vi "Main.vi"() -> ()   [LabVIEW 2019]
doc: "Main Program initialize config files, handles user inputs, image acquisition, object detection and image storing. User interface is handled in a state machine sending outputs."
uses:
  controls/State.ctl
  controls/Data.ctl
  <vilib>/userdefined/High Color/IMAQdx.ctl
  <vilib>/vision/Image Controls.llb/IMAQ Image.ctl
  b1a6e15a-21f6-4224-89c9-cebb1e441bce.vi
  4203ab90-da59-4329-829c-edbd02661f10.vi
  <extravilib>/ChannelInstances/Tag-bool/Read With Abort.vi
  <extravilib>/ChannelInstances/Tag-t'Data.ctl'/Read With Abort.vi
  <extravilib>/ChannelInstances/Tag-c(bool,bool)/Read With Abort.vi
  <extravilib>/ChannelInstances/Tag-c(bool,bool)/Write With Abort.vi
  <extravilib>/ChannelInstances/Tag-t'Data.ctl'/Write With Abort.vi
  <extravilib>/ChannelInstances/Tag-bool/Write With Abort.vi
  <extravilib>/ChannelInstances/Tag-c(bool,bool)/Instantiate.vi
  <extravilib>/ChannelInstances/Tag-t'Data.ctl'/Instantiate.vi
  <extravilib>/ChannelInstances/Tag-bool/Instantiate.vi
  <extravilib>/ChannelInstances/Tag-bool/EndpointRead.vi
  <extravilib>/ChannelInstances/Tag-t'Data.ctl'/EndpointRead.vi
  <extravilib>/ChannelInstances/Tag-c(bool,bool)/EndpointRead.vi
  <extravilib>/ChannelInstances/Tag-c(bool,bool)/Endpoint.vi
  <extravilib>/ChannelInstances/Tag-t'Data.ctl'/Endpoint.vi
  <extravilib>/ChannelInstances/Tag-bool/Endpoint.vi
  <extravilib>/ChannelInstances/Tag-bool.lvlib
  <extravilib>/ChannelInstances/Tag-t'Data.ctl'.lvlib
  <extravilib>/ChannelInstances/Tag-c(bool,bool).lvlib
panel:
  in  "Tab Control":T1(tab)
  in  "Exposure Time":dbl=1000.0
  in  "Exposure":enum32{"Item 0", "Item 1", "Item 2", "Item 3"}(radio)=enum."Item 3"
  in  "Aperture":enum32{"Item 0", "Item 1", "Item 2", "Item 3"}(radio)
  in  "Other notes":string caption="Sample Name"
  in  "Species Name":string="Test Sample" caption="Sample Name"
  in  "Station":string="Station" caption="Sample Name"
  in  "Collection date":string="24/06/2016" caption="Collection Date (DD/MM/YYYY)"
  out "Ready":bool
  in  "Operator":string="MRJ" caption="Sample Name"
  out "Active":bool
  in  "Start Image Capture":bool
  in  "Sample Name":string="#0000"
  in  "Stop Image Capture":bool
  in  "Calibration Pictures":bool
  out "Camera 2":bool
  out "Camear 1":bool
  out "Pump":bool
  out "Actuator":bool
  in  "Connect Systems":bool
  in  "Exit":bool
  in  "Empty and Refill":bool
  in  "Start System":bool
  in  "Empty System":bool
  out "Process queue":T2(graph)
  out "Image Saving":T2(graph)
  in  "Empty Cuvette":bool
  in  "Max large object threshold":i32=4 min=1
  in  "Change Crop":bool
  in  "DetectCrop":dbl=30.0 caption="Movement Detection size" format="%#_g %"
  in  "Sample size threshold":i32=500 min=1
  in  "New Sample timeout":i32=50 min=1
  out "Target framerate":i32=100
  in  "Light intensity":i32(slide)=100 min=1 max=100 scale=1.0..100.0 scale format="%.0f%"
  in  "Max Framerate":i32=100 min=1
  in  "Overload threshold":i32=50 min=1
  in  "Img Save Que Size":i32=100 caption="Image Save Queue Size" min=1
  in  "Img Proc Que Size":i32=200 caption="Image Processing Queue Size" min=1
  in  "Manual Close":bool
  in  "Manual Open":bool
  out "Current Position":string
  in  "Position":bool
  in  "Pump Cycle":bool
  in  "Pump Bottom":bool
  in  "Pump Top":bool
  in  "Pump Terminate":bool
  out "Framerate":i32 caption="Current Framerate"
  out "Camera 1":T3(plugin-control)
  out "Camera 2":T3(plugin-control)
  out "Camera 1 Detect":T3(plugin-control)
  out "Camera 2 Detect":T3(plugin-control)
  out "Camera 1 Binary":T3(plugin-control)
  out "Camera 2 Binary":T3(plugin-control)
  # "SRS Software - Version 1.2.0.1"
  # "Connections"
  # "Detection settings"
  # "Image capture settings"
  # "Buffer settings"
  # "Hatch control"
  # "Pump"
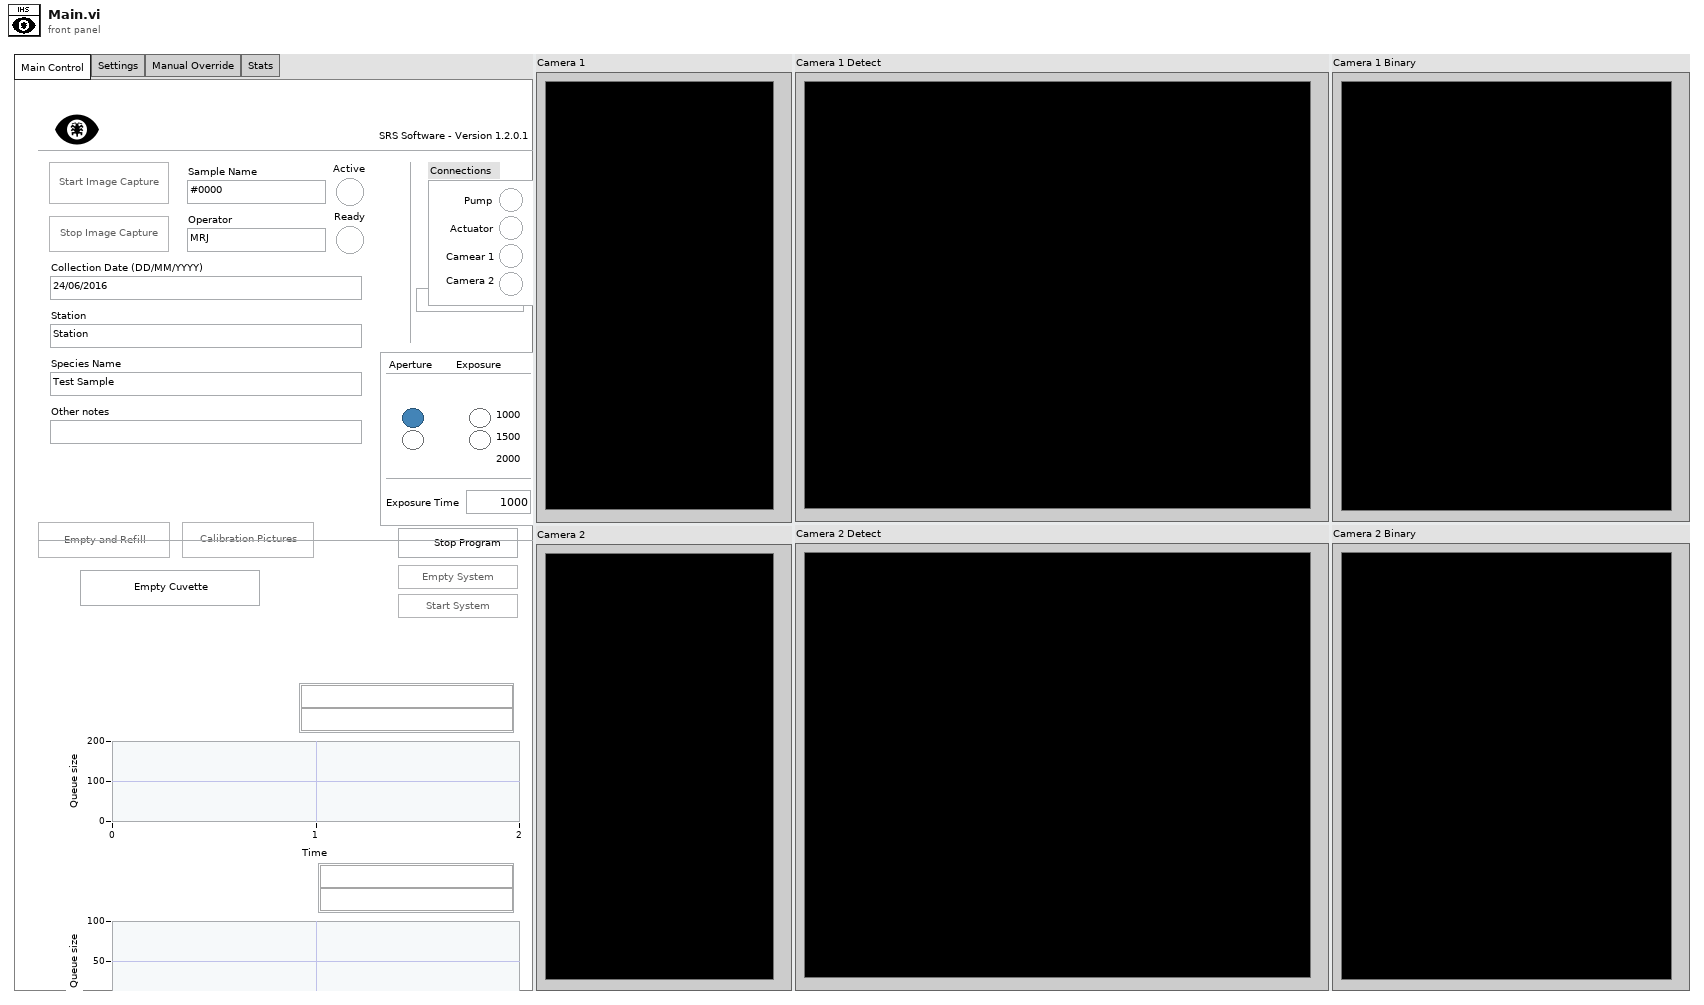
[diagram p1: front panel]
types:
  T1 = enum32{"Main Control", "Settings", "Manual Override", "Stats"}
  T2 = cluster{"# elements in queue":i32, "# elements in queue":i32}
  T3 = typedef "IMAQ Image.ctl" = refnum<image>
  T4 = typedef "Data.ctl" = cluster{"L16 Linear Actuator":refnum<visa-resource-name>, "XE 1000 Pump":refnum<visa-resource-name>, "Camera1":T5, "Camera2":T5, "Camera1_IMG":T3, "Camera2_IMG":T3, "Img_Capt":bool, "Actuator":bool, "Pump":bool, "Cam 1":bool, "Cam 2":bool, "Empty_Refill":bool, "Crop":bool, "Light intensity":i32, "Exposure Time":dbl, "Sample Name":string, "Operator":string, "Calibration 1":path, "Calibration 2":path, "Framerate":i32, "Timeout Sample":i32, "Collection date":string, "Sample size threshold":i32, "Empty start":u32, "Command":string, "Calibration Image 1":T3, "Calibration Image 2":T3, "Original Image 1":T3, "Original Image 2":T3, "Processing Image 1":T3, "Processing Image 2":T3, "Object Image 1":T3, "Object Image 2":T3, "Cam 1 - save queue":refnum<queue>, "Cam 2 - save queue":refnum<queue>, "Station":string, "Species Name":string, "Other Notes":string, "Aperture":enum32{"Item 0", "Item 1", "Item 2", "Item 3"}, "Image Process Queue Size":i32, "Image Save Queue Size":i32, "Overload threshold":i32, "Max Framerate":i32, "Blue Plane Image":T3, "Subtract Image":T3, "Binary Image 1":T3, "ROI mask allocation":T3, "Rectangle 1":T6, "Rectangle 2":T6, "Binary Image 2":T3, "Detection Region %":dbl, "Cam 1 queue":refnum<queue>, "Cam 2 queue":refnum<queue>, "Detect image 1":T3, "Detect image 2":T3, "Detect 1":path, "Detect 2":path, "Max large object threshold":i32, "Open(T)/Close(F)":bool}
  T5 = typedef "IMAQdx.ctl" = refnum<k21>
  T6 = typedef "IMAQ Rectangle" = cluster{"Left":i32, "Top":i32, "Right":i32, "Bottom":i32, "Rotation":dbl}
  T7 = typedef "State.ctl" = enum16{"Initialize", "Wait for Event", "Position", "Valve Signal", "Extra Flush", "Valve Cycle", "Valve Open", "Valve Close", "Pump Command", "Pump Cycle", "Empty System", "Start System", "Connect Systems", "Start Image Capture", "Stop Image Capture", "Calibration Pictures", "Empty and Refill", "Change Light Intensity", "Reconnect", "Exit"}
  T8 = enum8{"Enabled", "Disabled", "Disabled and Grayed Out"}
  T9 = cluster{"# elements in queue":i32, "# elements in queue":i32}[]
  T10 = typedef "Tag-t'Data.ctl'.lvlib/))Channel.ctl" = refnum<queue>
  T11 = typedef "Tag-bool.lvlib/))Channel.ctl" = refnum<queue>
  T12 = typedef "Tag-c(bool,bool).lvlib/))Channel.ctl" = refnum<queue>
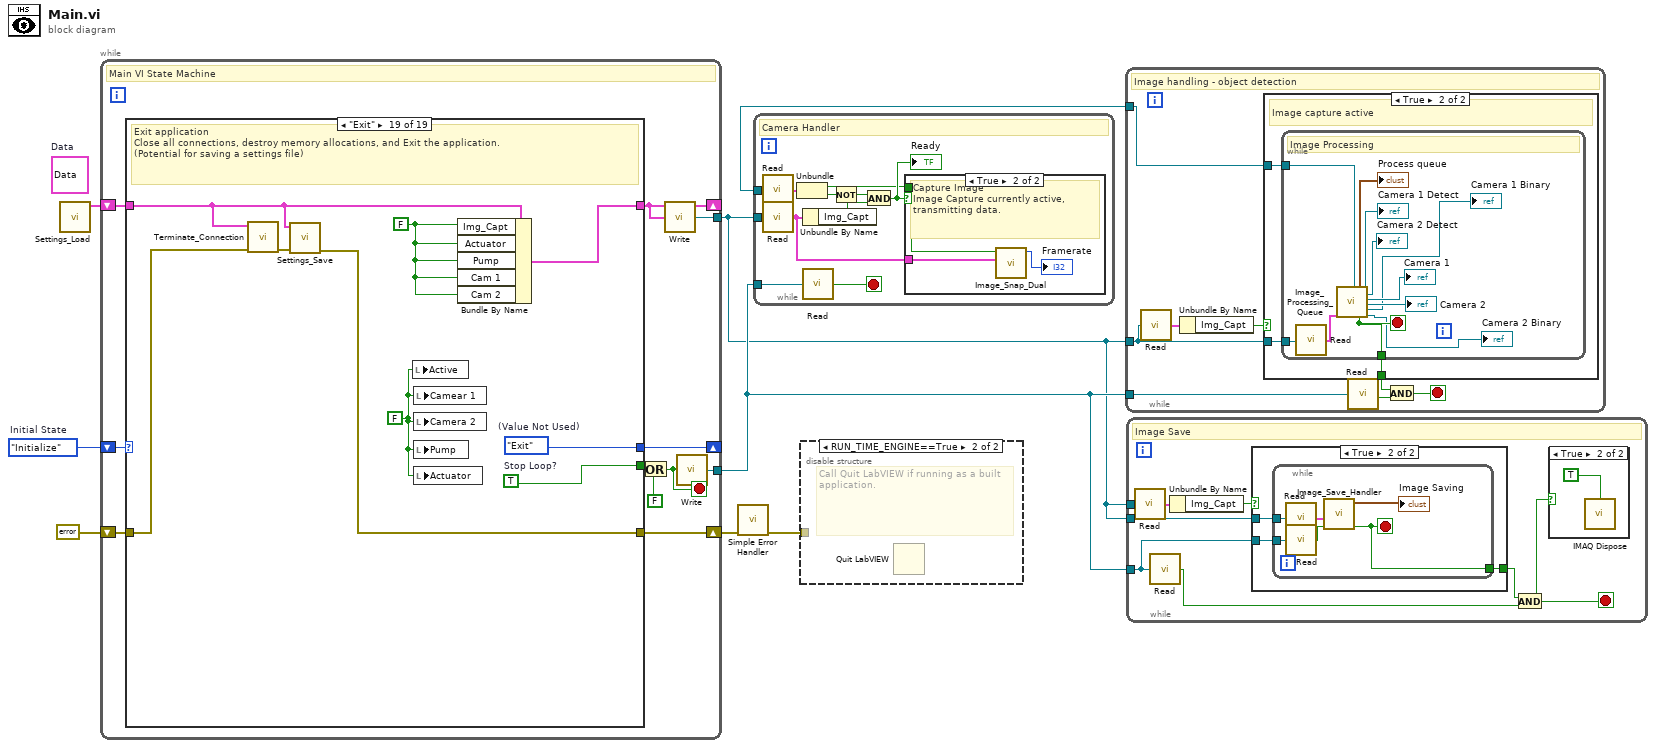
[diagram p0: block diagram]
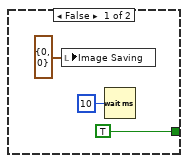
[diagram p3: hidden frame]
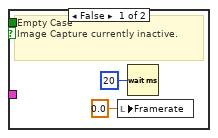
[diagram p4: hidden frame]
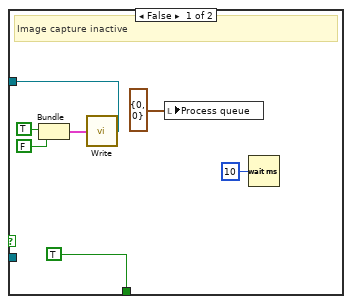
[diagram p5: hidden frame]
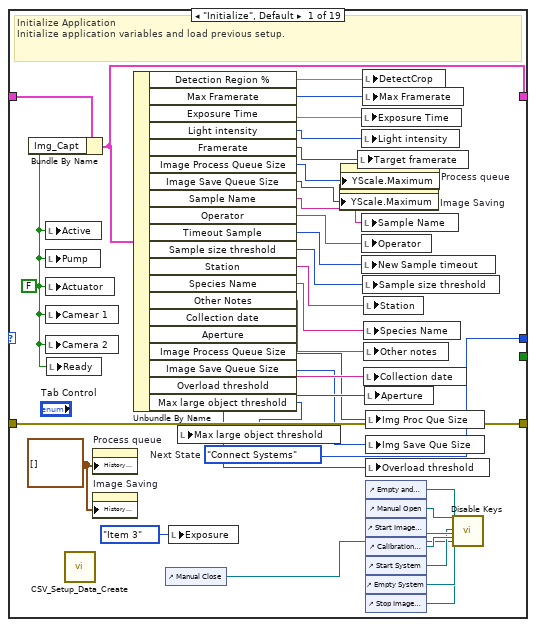
[diagram p7: hidden frame]
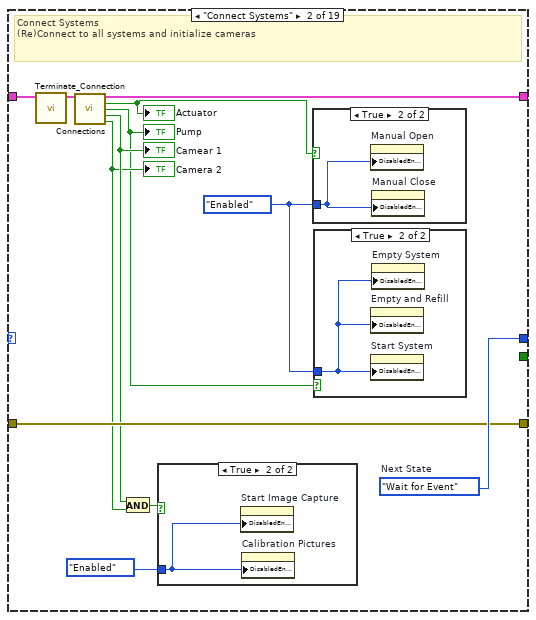
[diagram p8: hidden frame]
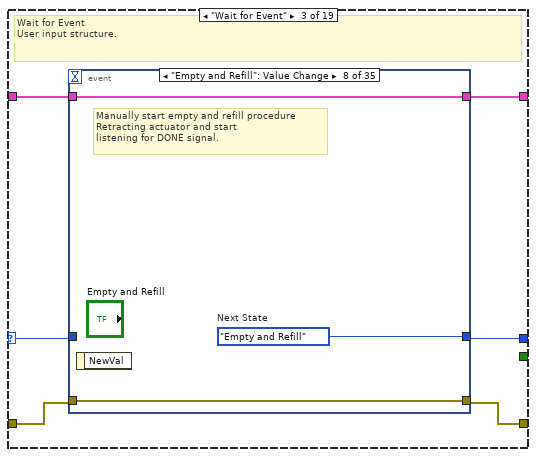
[diagram p12: hidden frame]
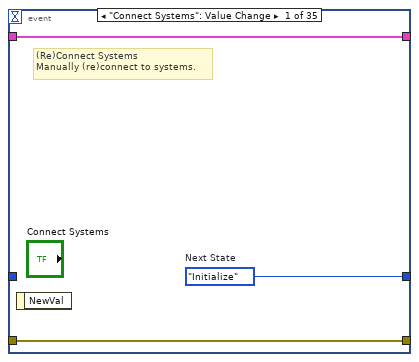
[diagram p13: hidden frame]
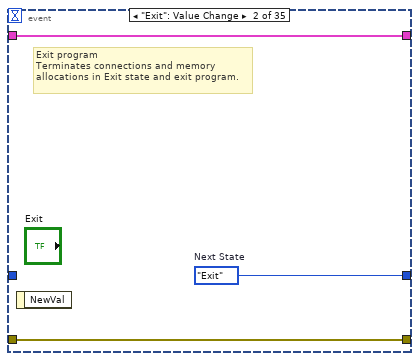
[diagram p14: hidden frame]
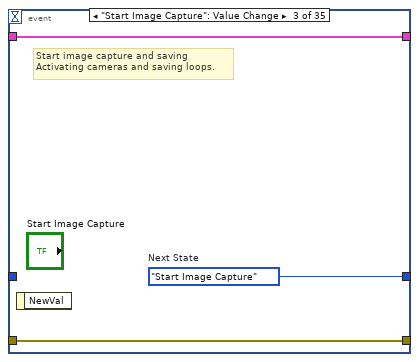
[diagram p15: hidden frame]
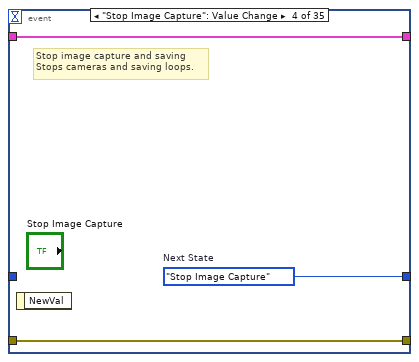
[diagram p16: hidden frame]
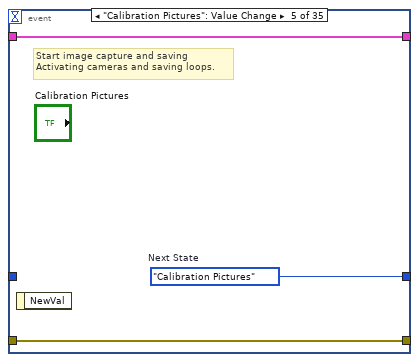
[diagram p17: hidden frame]
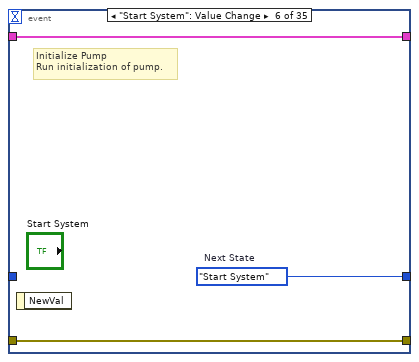
[diagram p18: hidden frame]
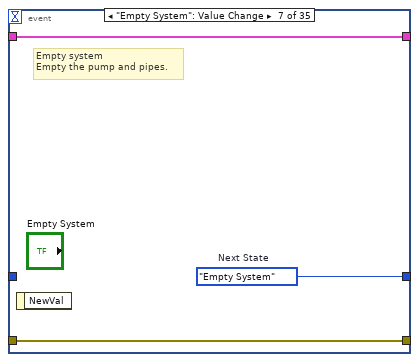
[diagram p19: hidden frame]
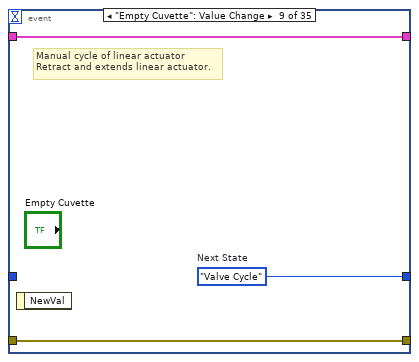
[diagram p20: hidden frame]
diagram:
  (unwired) T4 {"L16 Linear Actuator"="", "XE 1000 Pump"="", "Camera1"="", "Camera2"="", "Camera1_IMG"=refnum, "Camera2_IMG"=refnum, "Img_Capt"=FALSE, "Actuator"=FALSE, "Pump"=FALSE, "Cam 1"=FALSE, "Cam 2"=FALSE, "Empty_Refill"=FALSE, "Crop"=FALSE, "Light intensity"=100, "Exposure Time"=1000.0, "Sample Name"="Test Sample", "Operator"="MRJ", "Calibration 1"=path "C:/Users/au540322/Desktop/IHS_Project/images/Debris/Debris_0/Debris_0_2019_06_01-23-32-49-686.PNG", "Calibration 2"=path "C:/Users/au540322/Desktop/IHS_Project/images/Debris/Debris_0/Debris_0_2019_06_01-23-32-49-686.PNG", "Framerate"=100, "Timeout Sample"=200, "Collection date"="", "Sample size threshold"=500, "Empty start"=1, "Command"="", "Calibration Image 1"=refnum, "Calibration Image 2"=refnum, "Original Image 1"=refnum, "Original Image 2"=refnum, "Processing Image 1"=refnum, "Processing Image 2"=refnum, "Object Image 1"=refnum, "Object Image 2"=refnum, "Cam 1 - save queue"=refnum, "Cam 2 - save queue"=refnum, "Station"="", "Species Name"="", "Other Notes"="", "Aperture"=enum."Item 0", "Image Process Queue Size"=500, "Image Save Queue Size"=500, "Overload threshold"=500, "Max Framerate"=100, "Blue Plane Image"=refnum, "Subtract Image"=refnum, "Binary Image 1"=refnum, "ROI mask allocation"=refnum, "Rectangle 1"={"Left"=0, "Top"=0, "Right"=0, "Bottom"=0, "Rotation"=0.0}, "Rectangle 2"={"Left"=0, "Top"=0, "Right"=0, "Bottom"=0, "Rotation"=0.0}, "Binary Image 2"=refnum, "Detection Region %"=0.0, "Cam 1 queue"=refnum, "Cam 2 queue"=refnum, "Detect image 1"=refnum, "Detect image 2"=refnum, "Detect 1"=path "C:/Users/au540322/Desktop/IHS_Project/images/Debris/Debris_0/Debris_0_2019_06_01-23-32-49-686.PNG", "Detect 2"=path "C:/Users/au540322/Desktop/IHS_Project/images/Debris/Debris_0/Debris_0_2019_06_01-23-32-49-686.PNG", "Max large object threshold"=0, "Open(T)/Close(F)"=FALSE}  # Data
  w8 = State."Initialize"  # Initial State
  n1 = call "Settings_Load.vi"() -> ("value"=w4:T4)  [unwired: 10 in, 1 out]
  n2 = while {
    shift-right: [w18] -> _
    shift-left: w8 -> [w19]
    shift-right: [w16] -> _
    shift-left: w4 -> [w17]
    shift-right: [w13] -> w6
    shift-left: errorcluster {"status"=FALSE, "code"=0, "source"=""} ("error constant") -> [w15]
    tunnel: [w10] -> w3
    tunnel: [w11] -> w2
    stop <- w14 stop-if-true
    # "Main VI State Machine"
    n3 = case shown="\"Exit\"" w19 {
      selector: w19 -> [_ _ w70 _ _ _ _ _ _ _ _ _ _ _ _ _ _ _ _]
      tunnel: [w54 w66 w75 w253 w271 w288 w307 w313 w330 w347 w355 w368 w386 w393 w416 w428 w446 w449 w462] -> w18
      tunnel: [_ _ _ _ _ _ _ _ _ _ _ _ _ _ _ _ _ _ w461] -> w12
      tunnel: w17 -> [w46 w63 w74 w254 w267 w284 w301 w317 w334 w339 w353 w366 w385 w392 w415 w418 w430 w453 w455]
      tunnel: [w52 w64 w73 w255 w269 w274 w306 w308 w334 w340 w350 w365 w385 w392 w415 w417 w429 w453 w458] -> w16
      tunnel: w15 -> [w53 w65 w72 w256 w270 w287 w296 w316 w331 w345 w358 w370 w381 w389 w411 w425 w443 w452 w460]
      tunnel: [w53 w65 w71 w256 w270 w287 w289 w316 w324 w344 w356 w359 w380 w388 w410 w424 w434 w450 w454] -> w13
      frame "Initialize", Default {
        w45 = T9 [] ("History Data")
        w44 = FALSE ("Pump")
        w54 = State."Connect Systems"  # Next State
        # "Initialize Application\nInitialize application variables and load previous setup."
        n4 = Bundle By Name(cluster=w46, "Img_Capt"=w44) -> (w52:T4)
        n5 = local write "Active"(w44) -> ()
        n6 = local write "Pump"(w44) -> ()
        n7 = local write "Actuator"(w44) -> ()
        n8 = local write "Camear 1"(w44) -> ()
        n9 = local write "Camera 2"(w44) -> ()
        n10 = local write "Ready"(w44) -> ()
        n11 = call "CSV_Setup_Data_Create.vi"() -> ()  [unwired: 11 in, 1 out]
        n12 = property on="Process queue" class="WFChart (strict)"("History Data"=w45) -> ()  [unwired: 2 in, 2 out]
        n13 = property on="Image Saving" class="WFChart (strict)"("History Data"=w45) -> ()  [unwired: 2 in, 2 out]
        n14 = Unbundle By Name(w52) -> ("Detection Region %"=w23:dbl, "Max Framerate"=w24:i32, "Exposure Time"=w51:dbl, "Light intensity"=w50:i32, "Framerate"=w49:i32, "Image Process Queue Size"=w22:i32, "Image Save Queue Size"=w21:i32, "Sample Name"=w48:string, "Operator"=w47:string, "Timeout Sample"=w43:i32, "Sample size threshold"=w42:i32, "Station"=w41:string, "Species Name"=w40:string, "Other Notes"=w39:string, "Collection date"=w38:string, "Aperture"=w37:enum32{"Item 0", "Item 1", "Item 2", "Item 3"}, "Image Process Queue Size"=w36:i32, "Image Save Queue Size"=w35:i32, "Overload threshold"=w34:i32, "Max large object threshold"=w20:i32)
        n15 = control-ref of="Manual Close"() -> (w26:refnum<vi>)
        n16 = local write "Exposure"(enum32{"Item 0", "Item 1", "Item 2", "Item 3"}."Item 3" ("Exposure")) -> ()
        n17 = local write "Max large object threshold"(w20) -> ()
        n18 = property on="Image Saving" class="WFChart (strict)"("YScale.Maximum"=w21) -> ()  [unwired: 2 in, 2 out]
        n19 = property on="Process queue" class="WFChart (strict)"("YScale.Maximum"=w22) -> ()  [unwired: 2 in, 2 out]
        n20 = local write "Target framerate"(w49) -> ()
        n21 = local write "Exposure Time"(w51) -> ()
        n22 = local write "Light intensity"(w50) -> ()
        n23 = local write "Sample Name"(w48) -> ()
        n24 = local write "Operator"(w47) -> ()
        n25 = local write "New Sample timeout"(w43) -> ()
        n26 = local write "DetectCrop"(w23) -> ()
        n27 = local write "Max Framerate"(w24) -> ()
        n28 = local write "Sample size threshold"(w42) -> ()
        n29 = local write "Station"(w41) -> ()
        n30 = local write "Species Name"(w40) -> ()
        n31 = local write "Other notes"(w39) -> ()
        n32 = local write "Collection date"(w38) -> ()
        n33 = local write "Aperture"(w37) -> ()
        n34 = local write "Img Proc Que Size"(w36) -> ()
        n35 = local write "Img Save Que Size"(w35) -> ()
        n36 = local write "Overload threshold"(w34) -> ()
        n37 = control-ref of="Empty and Refill"() -> (w33:refnum<vi>)
        n38 = control-ref of="Manual Open"() -> (w32:refnum<vi>)
        n39 = control-ref of="Start Image Capture"() -> (w30:refnum<vi>)
        n40 = control-ref of="Calibration Pictures"() -> (w31:refnum<vi>)
        n41 = control-ref of="Start System"() -> (w29:refnum<vi>)
        n42 = control-ref of="Empty System"() -> (w28:refnum<vi>)
        n43 = control-ref of="Stop Image Capture"() -> (w27:refnum<vi>)
        n44 = call "Disable Keys.vi"("Boolean in"=w32, "Bool Refnum 6"=w33, "Bool Refnum 4"=w27, "Bool Refnum 7"=w29, "Bool Refnum 9"=w30, "Bool Refnum 2"=w31, "Bool Refnum 8"=w26, "Bool Refnum 3"=w28) -> ()  [unwired: 20 in]
      }
      frame "Connect Systems" {
        w55 = T8."Enabled" ("Disabled")
        w66 = State."Wait for Event"  # Next State
        # "Connect Systems\n(Re)Connect to all systems and initialize cameras"
        n45 = call "Terminate_Connection.vi"("Data"=w63) -> ("Data out"=w62:T4)  [unwired: 9 in, 1 out]
        n46 = call "Connections.vi"("input cluster"=w62) -> ("output cluster"=w64:T4, "Linear Actuator"=w61:bool, "Pump"=w57:bool, "Camear 1"=w59:bool, "Camera 2"=w58:bool)  [unwired: 10 in]
        "Pump" <- w57
        "Actuator" <- w61
        "Camera 2" <- w58
        "Camear 1" <- w59
        n47 = And(x=w59, y=w58) -> (x .and. y?=w60:bool)
        n48 = case shown="True" w60 {
          tunnel: T8."Enabled" ("Disabled") -> [_ w68]
          frame False {
          }
          frame True {
            n49 = property on="Start Image Capture" class="Bool"("DisabledEnum"=w68) -> ()  [unwired: 2 in, 2 out]
            n50 = property on="Calibration Pictures" class="Bool"("DisabledEnum"=w68) -> ()  [unwired: 2 in, 2 out]
          }
        }
        n51 = case shown="True" w61 {
          tunnel: w55 -> [_ w69]
          frame False {
          }
          frame True {
            n52 = property on="Manual Open" class="Bool"("DisabledEnum"=w69) -> ()  [unwired: 2 in, 2 out]
            n53 = property on="Manual Close" class="Bool"("DisabledEnum"=w69) -> ()  [unwired: 2 in, 2 out]
          }
        }
        n54 = case shown="True" w57 {
          tunnel: w55 -> [_ w67]
          frame False {
          }
          frame True {
            n55 = property on="Empty and Refill" class="Bool"("DisabledEnum"=w67) -> ()  [unwired: 2 in, 2 out]
            n56 = property on="Start System" class="Bool"("DisabledEnum"=w67) -> ()  [unwired: 2 in, 2 out]
            n57 = property on="Empty System" class="Bool"("DisabledEnum"=w67) -> ()  [unwired: 2 in, 2 out]
          }
        }
      }
      frame "Wait for Event" {
        # "Wait for Event\nUser input structure."
        n58 = event shown="[7] \"Empty and Refill\": Value Change" {
          selector: _ -> [_ _ _ _ _ _ _ _ _ _ _ _ _ _ _ _ _ _ _ _ _ _ _ _ _ _ _ _ _ _ _ _ _ _ _]
          dyn-events: _ -> [_ _ _ _ _ _ _ _ _ _ _ _ _ _ _ _ _ _ _ _ _ _ _ _ _ _ _ _ _ _ _ _ _ _ _]
          timeout: _ -> [_ _ _ _ _ _ _ _ _ _ _ _ _ _ _ _ _ _ _ _ _ _ _ _ _ _ _ _ _ _ _ _ _ _ _]
          tunnel: [w78 w81 w84 w87 w90 w93 w96 w99 w102 w105 w108 w111 w114 w119 w124 w129 w130 w135 State."Wait for Event" ("Next State") State."Wait for Event" ("Next State") State."Wait for Event" ("Next State") State."Wait for Event" ("Next State") State."Wait for Event" ("Next State") State."Wait for Event" ("Next State") State."Wait for Event" ("Next State") w197 w202 w207 w219 State."Change Light Intensity" ("Next State") w228 w233 State."Change Light Intensity" ("Next State") State."Wait for Event" ("Next State") w250] -> w75
          tunnel: w74 -> [w76 w80 w82 w85 w88 w91 w94 w97 w100 w103 w106 w109 w112 w116 w121 w126 w133 w136 w140 w146 w151 w156 w163 w168 w191 w198 w203 w208 w212 w225 w230 w235 w240 w245 w248]
          tunnel: [w76 w80 w82 w85 w88 w91 w94 w97 w100 w103 w106 w109 w112 w115 w120 w125 w132 w137 w141 w147 w152 w157 w160 w176 w192 w199 w204 w209 w220 w224 w229 w234 w239 w244 w247] -> w73
          tunnel: w72 -> [w77 w79 w83 w86 w89 w92 w95 w98 w101 w104 w107 w110 w113 w118 w123 w128 w134 w139 w144 w149 w154 w159 w165 w178 w195 w200 w205 w210 w221 w226 w231 w236 w241 w246 w249]
          tunnel: [w77 w79 w83 w86 w89 w92 w95 w98 w101 w104 w107 w110 w113 w118 w123 w128 w134 w139 w144 w149 w154 w159 w165 w178 w195 w200 w205 w210 w221 w226 w231 w236 w241 w246 w249] -> w71
          tunnel: w70 -> [_ _ _ _ _ _ _ _ _ _ _ _ _ _ _ _ _ _ _ _ _ _ _ _ _ _ _ _ _ _ _ _ _ _ _]
          event "Connect Systems": Value Change {
            w78 = State."Initialize"  # Next State
            # "(Re)Connect Systems\nManually (re)connect to systems."
            n59 = event-data() -> ()  [unwired: 1 in, 1 out]
          }
          event "Exit": Value Change {
            w81 = State."Exit"  # Next State
            # "Exit program\nTerminates connections and memory\nallocations in Exit state and exit program."
            n60 = event-data() -> ()  [unwired: 1 in, 1 out]
          }
          event "Start Image Capture": Value Change {
            w84 = State."Start Image Capture"  # Next State
            # "Start image capture and saving\nActivating cameras and saving loops."
            n61 = event-data() -> ()  [unwired: 1 in, 1 out]
          }
          event "Stop Image Capture": Value Change {
            w87 = State."Stop Image Capture"  # Next State
            # "Stop image capture and saving\nStops cameras and saving loops."
            n62 = event-data() -> ()  [unwired: 1 in, 1 out]
          }
          event "Calibration Pictures": Value Change {
            w90 = State."Calibration Pictures"  # Next State
            # "Start image capture and saving\nActivating cameras and saving loops."
            n63 = event-data() -> ()  [unwired: 1 in, 1 out]
          }
          event "Start System": Value Change {
            w93 = State."Start System"  # Next State
            # "Initialize Pump\nRun initialization of pump."
            n64 = event-data() -> ()  [unwired: 1 in, 1 out]
          }
          event "Empty System": Value Change {
            w96 = State."Empty System"  # Next State
            # "Empty system\nEmpty the pump and pipes."
            n65 = event-data() -> ()  [unwired: 1 in, 1 out]
          }
          event "Empty and Refill": Value Change {
            w99 = State."Empty and Refill"  # Next State
            # "Manually start empty and refill procedure\nRetracting actuator and start \nlistening for DONE signal."
            n66 = event-data() -> ()  [unwired: 1 in, 1 out]
          }
          event "Empty Cuvette": Value Change {
            w102 = State."Valve Cycle"  # Next State
            # "Manual cycle of linear actuator\nRetract and extends linear actuator."
            n67 = event-data() -> ()  [unwired: 1 in, 1 out]
          }
          event "Manual Open": Value Change {
            w105 = State."Valve Open"  # Next State
            # "Manual extend\nManually extend linear actuator."
            n68 = event-data() -> ()  [unwired: 1 in, 1 out]
          }
          event "Manual Close": Value Change {
            w108 = State."Valve Close"  # Next State
            # "Manual Retract\nManually retract linear actuator."
            n69 = event-data() -> ()  [unwired: 1 in, 1 out]
          }
          event "Position": Value Change {
            w111 = State."Position"  # Next State
            # "Read position\nRead linear actuator position."
            n70 = event-data() -> ()  [unwired: 1 in, 1 out]
          }
          event "Pump Cycle": Value Change {
            w114 = State."Pump Cycle"  # Next State
            # "Manual Pump Cycle\nManually go through a pump cycle."
            n71 = event-data() -> ()  [unwired: 1 in, 1 out]
          }
          event "Pump Top": Value Change {
            w119 = State."Pump Command"  # Next State
            # "Manual Move Pump Top\nManually move the pump \nto the top position."
            n72 = event-data() -> ()  [unwired: 1 in, 1 out]
            n73 = Bundle By Name(cluster=w116, "Command"="A1000R" ("write buffer 2")) -> (w115:T4)
          }
          event "Pump Bottom": Value Change {
            w124 = State."Pump Command"  # Next State
            # "Manual Move Pump Bottom\nManually move the pump\nto the bottom position."
            n74 = event-data() -> ()  [unwired: 1 in, 1 out]
            n75 = Bundle By Name(cluster=w121, "Command"="A0R" ("write buffer 2")) -> (w120:T4)
          }
          event "Pump Terminate": Value Change {
            w129 = State."Pump Command"  # Next State
            # "Terminate Pump\nAbort all current pump commands, \nacts as emergency stop."
            n76 = event-data() -> ()  [unwired: 1 in, 1 out]
            n77 = Bundle By Name(cluster=w126, "Command"="T" ("write buffer 2")) -> (w125:T4)
          }
          event "Sample Name": Value Change {
            w130 = State."Wait for Event"  # Next State
            # "Sample Name\nSample Name, used in image folders,\nand saved in sample information file."
            n78 = event-data() -> ()  [unwired: 1 in, 3 out]
            n79 = Bundle By Name(cluster=w133, "Sample Name"="Sample Name") -> (w132:T4)
          }
          event "Operator": Value Change {
            w135 = State."Wait for Event"  # Next State
            # "Operator Name\nOperator Name, saved in sample information file."
            n80 = event-data() -> ()  [unwired: 1 in, 3 out]
            n81 = Bundle By Name(cluster=w136, "Operator"="Operator") -> (w137:T4)
          }
          event "Collection date": Value Change {
            # "Sample Notes\nNotes/Description, saved in sample \ninformation file."
            n82 = event-data() -> ()  [unwired: 1 in, 3 out]
            n83 = Bundle By Name(cluster=w140, "Collection date"="Collection date") -> (w141:T4)
          }
          event "Station": Value Change {
            # "Sample Notes\nNotes/Description, saved in sample \ninformation file."
            n84 = event-data() -> ()  [unwired: 1 in, 3 out]
            n85 = Bundle By Name(cluster=w146, "Station"="Station") -> (w147:T4)
          }
          event "Species Name": Value Change {
            # "Sample Notes\nNotes/Description, saved in sample \ninformation file."
            n86 = event-data() -> ()  [unwired: 1 in, 3 out]
            n87 = Bundle By Name(cluster=w151, "Species Name"="Species Name") -> (w152:T4)
          }
          event "Other notes": Value Change {
            # "Sample Notes\nNotes/Description, saved in sample \ninformation file."
            n88 = event-data() -> ()  [unwired: 1 in, 3 out]
            n89 = Bundle By Name(cluster=w156, "Other Notes"="Other notes") -> (w157:T4)
          }
          event "Aperture": Value Change {
            # "Aperture\nAperture setting (manually changed on cameras)\nsaved in information file. Loads calibration image."
            n90 = event-data() -> ()  [unwired: 1 in, 3 out]
            n91 = Bundle By Name(cluster=w163, "Aperture"="Aperture") -> (w161:T4)
            n92 = call "Calibration_Update.vi"("value"=w161) -> ("output cluster"=w160:T4)  [unwired: 10 in]
          }
          event "Exposure": Value Change {
            n93 = event-data() -> ()  [unwired: 1 in, 3 out]
            n94 = Unbundle By Name(w168) -> ("Max Framerate"=w173:i32)
            n95 = case shown="\"Item 3\"" "Exposure" {
              tunnel: [1000.0 1500.0 2000.0 w182] -> w166
              frame "Item 0", Default {
              }
              frame "Item 1" {
              }
              frame "Item 2" {
              }
              frame "Item 3" {
                n96 = local read "Exposure Time"() -> (w182:dbl)
              }
            }
            n97 = Multiply(x=w166, y=10.0) -> (x*y=w171:dbl)
            n98 = Divide(x=1000000.0, y=w171) -> (x/y=w172:dbl)
            n99 = Max & Min(x=w172, y=w173) -> (min(x,y)=w174:dbl)  [unwired: 1 out]
            n100 = local write "Exposure Time"(w166) -> ()
            n101 = Bundle By Name(cluster=w168, "Exposure Time"=w166, "Framerate"=w174) -> (w167:T4)
            n102 = local write "Target framerate"(w174) -> ()
            n103 = call "Calibration_Update.vi"("value"=w167) -> ("output cluster"=w176:T4)  [unwired: 10 in]
          }
          event "Exposure Time": Value Change {
            # "Exposure Time\nChanges camera exposure time, must restart image\nacquisition to enable new value. Value is saved in \nsample information file."
            n104 = event-data() -> ()  [unwired: 1 in, 3 out]
            n105 = Unbundle By Name(w191) -> ("Max Framerate"=w185:i32)
            n106 = Multiply(x="Exposure Time", y=10.0) -> (x*y=w188:dbl)
            n107 = Divide(x=1000000.0, y=w188) -> (x/y=w186:dbl)
            n108 = Max & Min(x=w186, y=w185) -> (min(x,y)=w184:dbl)  [unwired: 1 out]
            "Target framerate" <- w184
            n109 = Bundle By Name(cluster=w191, "Exposure Time"="Exposure Time", "Framerate"=w184) -> (w193:T4)
            n110 = local write "Exposure"(enum32{"Item 0", "Item 1", "Item 2", "Item 3"}."Item 3" ("Exposure")) -> ()
            n111 = call "Calibration_Update.vi"("value"=w193) -> ("output cluster"=w192:T4)  [unwired: 10 in]
          }
          event "Img Proc Que Size": Value Change {
            w197 = State."Wait for Event"  # Next State
            # "Image Processing Queue Size\nMaximum buffer size of the image processing queue."
            n112 = event-data() -> ()  [unwired: 1 in, 3 out]
            n113 = Bundle By Name(cluster=w198, "Image Process Queue Size"="Img Proc Que Size") -> (w199:T4)
            n114 = property on="Process queue" class="WFChart (strict)"("YScale.Maximum"="Img Proc Que Size") -> ()  [unwired: 2 in, 2 out]
          }
          event "Img Save Que Size": Value Change {
            w202 = State."Wait for Event"  # Next State
            # "Image Save Queue Size\nMaximum buffer size of the image saving queue."
            n115 = event-data() -> ()  [unwired: 1 in, 3 out]
            n116 = Bundle By Name(cluster=w203, "Image Save Queue Size"="Img Save Que Size") -> (w204:T4)
            n117 = property on="Image Saving" class="WFChart (strict)"("YScale.Maximum"="Img Save Que Size") -> ()  [unwired: 2 in, 2 out]
          }
          event "Overload threshold": Value Change {
            w207 = State."Wait for Event"  # Next State
            # "Overload threshold (Image Processing)\nSet buffer size limit to overloading threshold. Values over this\nthreshold (while no object currently detected), will pause image\ncapture until image processing queue is empty."
            n118 = event-data() -> ()  [unwired: 1 in, 3 out]
            n119 = Bundle By Name(cluster=w208, "Overload threshold"="Overload threshold") -> (w209:T4)
          }
          event "Max Framerate": Value Change {
            w219 = State."Wait for Event"  # Next State
            # "Maximum Framerate\nMaximum image capture framerate."
            n120 = event-data() -> ()  [unwired: 1 in, 3 out]
            n121 = Unbundle By Name(w212) -> ("Exposure Time"=w217:dbl)
            n122 = Multiply(x=w217, y=10.0) -> (x*y=w216:dbl)
            n123 = Divide(x=1000000.0, y=w216) -> (x/y=w218:dbl)
            n124 = Max & Min(x="Max Framerate", y=w218) -> (min(x,y)=w211:dbl)  [unwired: 1 out]
            n125 = Bundle By Name(cluster=w212, "Max Framerate"="Max Framerate", "Framerate"=w211) -> (w220:T4)
            n126 = local write "Target framerate"(w211) -> ()
          }
          event "Light intensity": Value Change {
            # "Light Intensity\nChanges light intensity, value is  saved in \nsample information file."
            n127 = event-data() -> ()  [unwired: 1 in, 3 out]
            n128 = Bundle By Name(cluster=w225, "Light intensity"="Light intensity") -> (w224:T4)
          }
          event "New Sample timeout": Value Change {
            w228 = State."Wait for Event"  # Next State
            # "Framerate\nDefined the save frequency (saves every nth image)\nValue saved in sample information file."
            n129 = event-data() -> ()  [unwired: 1 in, 3 out]
            n130 = Bundle By Name(cluster=w230, "Timeout Sample"="New Sample timeout") -> (w229:T4)
          }
          event "Sample size threshold": Value Change {
            w233 = State."Wait for Event"  # Next State
            # "Framerate\nDefined the save frequency (saves every nth image)\nValue saved in sample information file."
            n131 = event-data() -> ()  [unwired: 1 in, 3 out]
            n132 = Bundle By Name(cluster=w235, "Sample size threshold"="Sample size threshold") -> (w234:T4)
          }
          event "Max large object threshold": Value Change {
            # "Array size threshold\nChanges array size threshold, used to check if too many,\nobjects currently detected."
            n133 = event-data() -> ()  [unwired: 1 in, 3 out]
            n134 = Bundle By Name(cluster=w240, "Max large object threshold"="Max large object threshold") -> (w239:T4)
          }
          event "DetectCrop": Value Change {
            # "Movement Detection Crop %\nChanges the percentage of the image used for detecting\nmovement, before full image is tracked."
            n135 = event-data() -> ()  [unwired: 1 in, 3 out]
            n136 = Bundle By Name(cluster=w245, "Detection Region %"="DetectCrop") -> (w244:T4)
          }
          event "Change Crop": Value Change {
            w250 = State."Wait for Event"  # Next State
            # "Change crop\nChange the cropping of images."
            n137 = event-data() -> ()  [unwired: 1 in, 1 out]
            n138 = call "Camera_Crop_Setup.vi"("value"=w248) -> ("output cluster"=w247:T4)  [unwired: 10 in]
          }
        }
      }
      frame "Start Image Capture" {
        # "Start Image Capture\nActivating Camera and Image saving loops."
        n139 = call "Calibration_Load.vi"("Data in"=w254) -> ("Next State"=w253:T7, "Calibration error?"=w251:bool, "Data out"=w252:T4)  [unwired: 8 in]
        n140 = case shown="False" w251 {
          tunnel: [w261 w263] -> w255
          tunnel: w252 -> [w258 w263]
          frame False {
            # "Calibration image\nloaded succesfully."
            n141 = call "Capture_Save_Initialize.vi"("input cluster"=w258) -> ("output cluster"=w261:T4)  [unwired: 10 in]
            n142 = property on="Stop Image Capture" class="Bool"("DisabledEnum"=T8."Enabled" ("Disabled")) -> ()  [unwired: 2 in, 2 out]
            n143 = property on="Start Image Capture" class="Bool"("DisabledEnum"=T8."Disabled and Grayed Out" ("Disabled")) -> ()  [unwired: 2 in, 2 out]
            n144 = property on="Calibration Pictures" class="Bool"("DisabledEnum"=T8."Disabled and Grayed Out" ("Disabled")) -> ()  [unwired: 2 in, 2 out]
            "Active" <- TRUE ("Image_Capture")
          }
          frame True {
            # "Error loading calibration."
          }
        }
      }
      frame "Stop Image Capture" {
        w265 = T8."Enabled" ("Disabled")
        w268 = FALSE ("Image_Capture")
        w271 = State."Wait for Event"  # Next State
        # "Stop Image Capture\nStopping Camera and Image saving loops."
        n145 = call "Image_Acquisition_Stop.vi"("input cluster"=w267) -> ("Output cluster"=w264:T4)  [unwired: 10 in]
        n146 = Bundle By Name(cluster=w264, "Img_Capt"=w268) -> (w269:T4)
        n147 = local write "Active"(w268) -> ()
        n148 = property on="Start Image Capture" class="Bool"("DisabledEnum"=w265) -> ()  [unwired: 2 in, 2 out]
        n149 = property on="Calibration Pictures" class="Bool"("DisabledEnum"=w265) -> ()  [unwired: 2 in, 2 out]
        n150 = property on="Stop Image Capture" class="Bool"("DisabledEnum"=T8."Disabled and Grayed Out" ("Disabled")) -> ()  [unwired: 2 in, 2 out]
      }
      frame "Calibration Pictures" {
        w288 = State."Wait for Event"  # Next State
        # "Start Image Capture\nTake two calibration pictures with each camera and save in calibration folder."
        n151 = call "Calibration_Capture.vi"("Crop?"=FALSE, "value"=w284) -> ("Image2"=w281:T3, "Image1"=w282:T3, "output cluster"=w283:T4)  [unwired: 7 in]
        n152 = local write "Camera 2"(w281) -> ()
        n153 = local write "Camera 1"(w282) -> ()
        n154 = call "Calibration_Capture.vi"("Detect Movement"=FALSE, "Crop?"=TRUE, "value"=w283) -> ("Image2"=w279:T3, "Image1"=w280:T3, "output cluster"=w275:T4)  [unwired: 6 in]
        n155 = local write "Camera 2"(w279) -> ()
        n156 = local write "Camera 1"(w280) -> ()
        n157 = call "Calibration_Capture.vi"("Detect Movement"=TRUE, "Crop?"=TRUE, "value"=w275) -> ("Image2"=w272:T3, "Image1"=w273:T3, "output cluster"=w274:T4)  [unwired: 6 in]
        n158 = local write "Camera 1"(w273) -> ()
        n159 = local write "Camera 2"(w272) -> ()
      }
      frame "Empty and Refill" {
        w299 = T8."Enabled" ("Disabled")
        w297 = TRUE ("Empty_Refill")
        w303 = FALSE ("Image_Capture")
        w307 = State."Valve Signal"  # Next State
        # "Empty and Refill command\nActivate Empty and refill of cuvette, start listening for valve return signal."
        n160 = Unbundle By Name(w301) -> ("XE 1000 Pump"=w291:refnum<visa-resource-name>, "L16 Linear Actuator"=w304:refnum<visa-resource-name>)
        n161 = VISA Write(VISA resource name=w304, write buffer="102", error in (no error)=w296) -> (error out=w290:errorcluster)  [unwired: 2 out]
        n162 = Concatenate Strings("/1IS20A200R" ("write buffer 2"), "\r\n") -> (w294:string)
        n163 = property on="Empty and Refill" class="Bool"("DisabledEnum"=T8."Disabled and Grayed Out" ("Disabled")) -> ()  [unwired: 2 in, 2 out]
        n164 = property on="Stop Image Capture" class="Bool"("DisabledEnum"=T8."Disabled and Grayed Out" ("Disabled")) -> ()  [unwired: 2 in, 2 out]
        n165 = property on="Start Image Capture" class="Bool"("DisabledEnum"=w299) -> ()  [unwired: 2 in, 2 out]
        n166 = property on="Calibration Pictures" class="Bool"("DisabledEnum"=w299) -> ()  [unwired: 2 in, 2 out]
        n167 = VISA Write(VISA resource name=w291, write buffer=w294, error in (no error)=w290) -> (error out=w289:errorcluster)  [unwired: 2 out]
        n168 = call "Image_Acquisition_Stop.vi"("input cluster"=w301) -> ("Output cluster"=w295:T4)  [unwired: 10 in]
        n169 = Tick Count (ms)() -> (millisecond timer value=w298:u32)
        n170 = Bundle By Name(cluster=w295, "Img_Capt"=w303, "Empty_Refill"=w297, "Open(T)/Close(F)"=w297, "Empty start"=w298) -> (w306:T4)
        n171 = local write "Active"(w303) -> ()
      }
      frame "Valve Signal" {
        # "Listen for valve return signal\nListen for valve return signal indicating valve is OPEN or CLOSED."
        n172 = call "Empty_Complete.vi"("input cluster"=w317) -> ("Next State"=w313:T7, "output cluster"=w308:T4)  [unwired: 9 in]
        n173 = local read "Pump"() -> (w309:bool)
        n174 = Equal?(x=State."Pump Cycle" ("Next State"), y=w313) -> (x = y?=w312:bool)
        n175 = Equal?(x=w313, y=State."Wait for Event" ("Next State")) -> (x = y?=w311:bool)
        n176 = Or(x=w312, y=w311) -> (x .or. y?=w310:bool)
        n177 = case shown="True" w310 {
          tunnel: w309 -> [_ w319]
          frame False {
          }
          frame True {
            w318 = T8."Enabled" ("Disabled")
            n178 = case shown="True" w319 {
              frame False {
              }
              frame True {
                n179 = property on="Empty and Refill" class="Bool"("DisabledEnum"=T8."Enabled" ("Disabled")) -> ()  [unwired: 2 in, 2 out]
              }
            }
            n180 = property on="Start Image Capture" class="Bool"("DisabledEnum"=w318) -> ()  [unwired: 2 in, 2 out]
            n181 = property on="Empty Cuvette" class="Bool"("DisabledEnum"=w318) -> ()  [unwired: 2 in, 2 out]
            n182 = property on="Calibration Pictures" class="Bool"("DisabledEnum"=w318) -> ()  [unwired: 2 in, 2 out]
          }
        }
      }
      frame "Position" {
        w330 = State."Wait for Event"  # Next State
        # "Read linear actuator position\nSend command and read linear actuator position."
        n183 = Unbundle By Name(w334) -> ("L16 Linear Actuator"=w333:refnum<visa-resource-name>)
        n184 = VISA Write(VISA resource name=w333, write buffer="104", error in (no error)=w331) -> (VISA resource name out=w323:refnum<visa-resource-name>, error out=w329:errorcluster)  [unwired: 1 out]
        n185 = call "Stall Data Flow.vim"("value in"=w323, "milliseconds to wait"=u32 500) -> ("value out"=w321:refnum<visa-resource-name>)  [unwired: 1 out]
        n186 = property class="Instr"(reference=w321, error in=w329) -> (reference out=w327:refnum<visa-resource-name>, error out=w326:errorcluster, "Serial Settings:Number of Bytes at Serial Port"=w328:u32)
        n187 = VISA Read(VISA resource name=w327, byte count=w328, error in (no error)=w326) -> (read buffer=→"Current Position":string, error out=w324:errorcluster)  [unwired: 2 out]
      }
      frame "Valve Cycle" {
        w338 = T8."Enabled" ("Disabled")
        w337 = T8."Disabled and Grayed Out" ("Disabled")
        w341 = FALSE ("Image_Capture")
        w347 = State."Valve Signal"  # Next State
        # "Manual cycle of linear actuator\nRetract and extend linear actuator."
        n188 = Unbundle By Name(w339) -> ("L16 Linear Actuator"=w346:refnum<visa-resource-name>)
        n189 = VISA Write(VISA resource name=w346, write buffer="102", error in (no error)=w345) -> (error out=w344:errorcluster)  [unwired: 2 out]
        n190 = property on="Start Image Capture" class="Bool"("DisabledEnum"=w338) -> ()  [unwired: 2 in, 2 out]
        n191 = property on="Calibration Pictures" class="Bool"("DisabledEnum"=w338) -> ()  [unwired: 2 in, 2 out]
        n192 = property on="Stop Image Capture" class="Bool"("DisabledEnum"=w337) -> ()  [unwired: 2 in, 2 out]
        n193 = property on="Empty Cuvette" class="Bool"("DisabledEnum"=w337) -> ()  [unwired: 2 in, 2 out]
        n194 = call "Image_Acquisition_Stop.vi"("input cluster"=w339) -> ("Output cluster"=w336:T4)  [unwired: 10 in]
        n195 = Tick Count (ms)() -> (millisecond timer value=w342:u32)
        n196 = Bundle By Name(cluster=w336, "Open(T)/Close(F)"=TRUE, "Img_Capt"=w341, "Empty_Refill"=w341, "Empty start"=w342) -> (w340:T4)
      }
      frame "Valve Open" {
        w355 = State."Wait for Event"  # Next State
        w349 = T8."Disabled and Grayed Out" ("Disabled")
        # "Manual extend of linear actuator\nSend extend command to linear actuator."
        n197 = Unbundle By Name(w353) -> ("L16 Linear Actuator"=w357:refnum<visa-resource-name>)
        n198 = VISA Write(VISA resource name=w357, write buffer="102", error in (no error)=w358) -> (error out=w356:errorcluster)  [unwired: 2 out]
        n199 = property on="Calibration Pictures" class="Bool"("DisabledEnum"=w349) -> ()  [unwired: 2 in, 2 out]
        n200 = property on="Start Image Capture" class="Bool"("DisabledEnum"=w349) -> ()  [unwired: 2 in, 2 out]
        n201 = property on="Stop Image Capture" class="Bool"("DisabledEnum"=w349) -> ()  [unwired: 2 in, 2 out]
        n202 = call "Image_Acquisition_Stop.vi"("input cluster"=w353) -> ("Output cluster"=w351:T4)  [unwired: 10 in]
        n203 = Bundle By Name(cluster=w351, "Img_Capt"=FALSE ("Image_Capture"), "Open(T)/Close(F)"=TRUE) -> (w350:T4)
      }
      frame "Valve Close" {
        w368 = State."Valve Signal"  # Next State
        # "Manual retract of linear actuator\nSend retract command to linear actuator."
        n204 = Unbundle By Name(w366) -> ("Empty_Refill"=w362:bool, "XE 1000 Pump"=w360:refnum<visa-resource-name>, "L16 Linear Actuator"=w369:refnum<visa-resource-name>)
        n205 = VISA Write(VISA resource name=w369, write buffer="101", error in (no error)=w370) -> (error out=w361:errorcluster)  [unwired: 2 out]
        n206 = case shown="True" w362 {
          tunnel: w361 -> [w371 w377]
          tunnel: w360 -> [_ w376]
          tunnel: [w371 w372] -> w359
          frame False {
            # "Manual Close, don't load volume."
          }
          frame True {
            # "Load specified volume in pump."
            n207 = Concatenate Strings("/1IS20A810R" ("write buffer 2"), "\r\n") -> (w373:string)
            n208 = VISA Write(VISA resource name=w376, write buffer=w373, error in (no error)=w377) -> (error out=w372:errorcluster)  [unwired: 2 out]
          }
        }
        n209 = Tick Count (ms)() -> (millisecond timer value=w364:u32)
        n210 = Bundle By Name(cluster=w366, "Empty start"=w364, "Open(T)/Close(F)"=FALSE) -> (w365:T4)
      }
      frame "Pump Command" {
        w386 = State."Wait for Event"  # Next State
        # "<I> Input valve\n<A> Absolute position (n = 1...1000)\n<O> Output valve\n<R> Execute commands\n<T> Abort commands"
        # "Pump command\nSend command to XE 1000 Pump."
        n211 = Unbundle By Name(w385) -> ("XE 1000 Pump"=w382:refnum<visa-resource-name>, "Command"=w379:string)
        n212 = Concatenate Strings("/1" ("string"), w379, "\r\n") -> (w383:string)
        n213 = VISA Write(VISA resource name=w382, write buffer=w383, error in (no error)=w381) -> (error out=w380:errorcluster)  [unwired: 2 out]
      }
      frame "Pump Cycle" {
        w393 = State."Wait for Event"  # Next State
        # "<I> Input valve\n<A> Absolute position (n = 1...1000)\n<O> Output valve\n<R> Execute commands\n<T> Abort commands"
        # "Pump Cycle\nSend command to XE 1000 Pump going through full cycle."
        n214 = Unbundle By Name(w392) -> ("Empty_Refill"=w391:bool, "XE 1000 Pump"=w390:refnum<visa-resource-name>)
        n215 = case shown="False" w391 {
          tunnel: w390 -> [w400 w407]
          tunnel: w389 -> [w396 w403]
          tunnel: [w395 w402] -> w388
          tunnel: [u32 5000 ("milliseconds to wait") u32 8500 ("milliseconds to wait")] -> w387
          frame True {
            # "Dispense ready volume."
            n216 = Concatenate Strings("/1S60OA0R" ("write buffer 2"), "\r\n") -> (w397:string)
            n217 = VISA Write(VISA resource name=w400, write buffer=w397, error in (no error)=w396) -> (error out=w395:errorcluster)  [unwired: 2 out]
          }
          frame False {
            # "Load and dispense volume."
            n218 = Concatenate Strings("/1IS20A810S60OA0R" ("write buffer 2"), "\r\n") -> (w404:string)
            n219 = VISA Write(VISA resource name=w407, write buffer=w404, error in (no error)=w403) -> (error out=w402:errorcluster)  [unwired: 2 out]
          }
        }
        n220 = Wait (ms)(milliseconds to wait=w387) -> ()  [unwired: 1 out]
      }
      frame "Extra Flush" {
        w416 = State."Valve Close"  # Next State
        # "<I> Input valve\n<A> Absolute position (n = 1...1000)\n<O> Output valve\n<R> Execute commands\n<T> Abort commands"
        # "Pump Extra Flush\nSend command to XE 1000 Pump dispensing an extra flush to clean Cuvette"
        n221 = Unbundle By Name(w415) -> ("XE 1000 Pump"=w412:refnum<visa-resource-name>)
        n222 = Concatenate Strings("/1S60OA0R" ("write buffer 2"), "\r\n") -> (w413:string)
        n223 = VISA Write(VISA resource name=w412, write buffer=w413, error in (no error)=w411) -> (error out=w410:errorcluster)  [unwired: 2 out]
        n224 = Wait (ms)(milliseconds to wait=u32 2000) -> ()  [unwired: 1 out]
      }
      frame "Start System" {
        w428 = State."Empty and Refill"  # Next State
        # "Y<n>: Initialize (Right input, Left output)  (<n> = speed 2-20 sec/stroke)\nS:<n>: Set speed (<n> = 20..600 strokes in 1/10 sec).\nA<n>: Absolute position (<n> = 1...1000)\nI: Input valve\nO: Output valve\nR: Execute commands\nT: Abort commands"
        # "Pump Initialize\nInitialize XE 1000 Pump and fill tubes, emptying cuvette and refill to full."
        n225 = Unbundle By Name(w418) -> ("XE 1000 Pump"=w426:refnum<visa-resource-name>)
        n226 = Concatenate Strings("/1Y5IS20A810S60OA0R" ("string"), "\r\n") -> (w427:string)
        n227 = VISA Write(VISA resource name=w426, write buffer=w427, error in (no error)=w425) -> (error out=w424:errorcluster)  [unwired: 2 out]
        n228 = Wait (ms)(milliseconds to wait=u32 10000) -> ()  [unwired: 1 out]
        n229 = property on="Empty and Refill" class="Bool"("DisabledEnum"=T8."Enabled" ("Disabled")) -> ()  [unwired: 2 in, 2 out]
        n230 = Bundle By Name(cluster=w418, "Img_Capt"=FALSE) -> (w417:T4)
      }
      frame "Empty System" {
        w446 = State."Valve Cycle"  # Next State
        # "<I> Input valve\n<A> Absolute position (n = 1...1000)\n<O> Output valve\n<R> Execute commands\n<T> Abort commands"
        # "Empty pump and pipes\nSend command to XE 1000 Pump and empty system."
        n231 = Unbundle By Name(w430) -> ("XE 1000 Pump"=w444:refnum<visa-resource-name>)
        n232 = Concatenate Strings("/1OS20A1000IA0" ("write buffer 2"), "OS20A1000IA0" ("write buffer 2"), "R" ("write buffer 2")) -> (w439:string)
        n233 = Concatenate Strings(w439, "\r\n") -> (w433:string)
        n234 = VISA Write(VISA resource name=w444, write buffer=w433, error in (no error)=w443) -> (VISA resource name out=w438:refnum<visa-resource-name>, error out=w435:errorcluster)  [unwired: 1 out]
        n235 = property on="Empty and Refill" class="Bool"("DisabledEnum"=T8."Disabled and Grayed Out" ("Disabled")) -> ()  [unwired: 2 in, 2 out]
        n236 = call "Stall Data Flow.vim"("value in"=w438, "milliseconds to wait"=u32 10000) -> ("value out"=w437:refnum<visa-resource-name>)  [unwired: 1 out]
        n237 = VISA Write(VISA resource name=w437, write buffer=w433, error in (no error)=w435) -> (error out=w434:errorcluster)  [unwired: 2 out]
        n238 = Bundle By Name(cluster=w430, "Img_Capt"=FALSE) -> (w429:T4)
      }
      frame "Change Light Intensity" {
        w449 = State."Wait for Event"  # Next State
        # "Manual extend of linear actuator\nSend extend command to linear actuator."
        n239 = Unbundle By Name(w453) -> ("L16 Linear Actuator"=w451:refnum<visa-resource-name>, "Light intensity"=w448:i32)
        n240 = Number To Decimal String(number=w448) -> (decimal integer string=w447:string)  [unwired: 1 in]
        n241 = VISA Write(VISA resource name=w451, write buffer=w447, error in (no error)=w452) -> (error out=w450:errorcluster)  [unwired: 2 out]
      }
      frame "Exit" {
        w457 = FALSE ("Pump")
        w459 = FALSE ("Pump")
        w461 = TRUE  # Stop Loop?
        w462 = State."Exit"  # (Value Not Used)
        # "Exit application\nClose all connections, destroy memory allocations, and Exit the application. \n(Potential for saving a settings file)"
        n242 = call "Terminate_Connection.vi"("error in"=w460, "Data"=w455) -> ("error out"=w456:errorcluster)  [unwired: 8 in, 1 out]
        n243 = call "Settings_Save.vi"("error in"=w456, "input cluster"=w455) -> ("error out"=w454:errorcluster)  [unwired: 9 in]
        n244 = local write "Active"(w459) -> ()
        n245 = local write "Camear 1"(w459) -> ()
        n246 = local write "Camera 2"(w459) -> ()
        n247 = local write "Pump"(w459) -> ()
        n248 = local write "Actuator"(w459) -> ()
        n249 = Bundle By Name(cluster=w455, "Img_Capt"=w457, "Actuator"=w457, "Pump"=w457, "Cam 1"=w457, "Cam 2"=w457) -> (w458:T4)
      }
    }
    n250 = Or(x=w12, y=FALSE) -> (x .or. y?=w14:bool)
    n251 = call <extravilib>:"Write.vi"("element"=w16) -> ("channel"=w11:T10)  [unwired: 1 out]
    n252 = call <extravilib>:"Write.vi"("element"=w14) -> ("channel"=w10:T11)  [unwired: 1 out]
  }
  n253 = call <vilib>:"Simple Error Handler.vi"("error in (no error)"=w6) -> ("error out"=w5:errorcluster)  [unwired: 4 in, 4 out]
  n254 = disable-structure shown="RUN_TIME_ENGINE==True" {
    disable-tunnel: w5 -> [_ _]
    frame condition #0 (active) {
    }
    frame condition #1 {
      # "Call Quit LabVIEW if running as a built application."
      n255 = Quit LabVIEW() -> ()  [unwired: 1 in]
    }
  }
  n256 = while {
    tunnel: w3 -> [w464]
    tunnel: w2 -> [w468]
    tunnel: [w463] -> w1
    stop <- w470 stop-if-true
    # "Image handling - object detection"
    n257 = call <extravilib>:"Read.vi"("channel"=w468) -> ("element"=w466:T4)  [unwired: 1 in, 1 out]
    n258 = Unbundle By Name(w466) -> ("Img_Capt"=w467:bool)
    n259 = case shown="True" w467 {
      tunnel: [TRUE ("Last Image?") w479] -> w469
      tunnel: w468 -> [_ w480]
      tunnel: [w473 w478] -> w463
      frame False {
        # "Image capture inactive"
        n260 = Bundle(TRUE, FALSE) -> (w474:cluster{bool, bool})  [unwired: 1 in]
        n261 = call <extravilib>:"Write.vi"("element"=w474) -> ("channel"=w473:T12)  [unwired: 1 out]
        n262 = local write "Process queue"(T2 {"# elements in queue"=0, "# elements in queue"=0} ("Image processing")) -> ()
        n263 = Wait (ms)(milliseconds to wait=u32 10) -> ()  [unwired: 1 out]
      }
      frame True {
        # "Image capture active"
        n264 = while "Save image" {
          tunnel: w480 -> [w486]
          tunnel: [w487] -> w479
          tunnel: [w481] -> w478
          stop <- w487 stop-if-true
          # "Image Processing"
          n265 = call <extravilib>:"Read.vi"("channel"=w486) -> ("element"=w485:T4)  [unwired: 1 in, 1 out]
          n266 = call "Image_Processing_Queue.vi"("Data"=w485) -> ("Status"=w481:T12, "Process queue"=→"Process queue":T2, "Last Image?"=w487:bool, "Object1"=→"Camera 1 Detect":T3, "Object2"=→"Camera 2 Detect":T3, "Image 1"=→"Camera 1":T3, "Image 2"=→"Camera 2":T3, "Binary 1"=→"Camera 1 Binary":T3, "Binary 2"=→"Camera 2 Binary":T3)  [unwired: 10 in]
        }
      }
    }
    n267 = call <extravilib>:"Read.vi"("channel"=w464) -> ("element"=w465:bool)  [unwired: 1 in, 1 out]
    n268 = And(x=w469, y=w465) -> (x .and. y?=w470:bool)
  }
  n269 = while {
    tunnel: w3 -> [w502]
    tunnel: w2 -> [w501]
    tunnel: w1 -> [w495]
    stop <- w499 stop-if-true
    # "Camera Handler"
    n270 = call <extravilib>:"Read.vi"("channel"=w495) -> ("element"=w494:cluster{bool, bool})  [unwired: 1 in, 1 out]
    n271 = call <extravilib>:"Read.vi"("channel"=w501) -> ("element"=w500:T4)  [unwired: 1 in, 1 out]
    n272 = Unbundle(w494) -> (w492:bool, w493:bool)
    n273 = Unbundle By Name(w500) -> ("Img_Capt"=w497:bool)
    n274 = call <extravilib>:"Read.vi"("channel"=w502) -> ("element"=w499:bool)  [unwired: 1 in, 1 out]
    n275 = Not(x=w493) -> (.not. x?=w498:bool)
    n276 = And(x=w498, y=w497) -> (x .and. y?=w496:bool)
    "Ready" <- w496
    n277 = case shown="True" w496 {
      tunnel: w500 -> [_ w506]
      tunnel: w492 -> [_ w505]
      frame False {
        # "Empty Case\nImage Capture currently inactive."
        n278 = local write "Framerate"(0.0 ("Framerate")) -> ()
        n279 = Wait (ms)(milliseconds to wait=u32 20) -> ()  [unwired: 1 out]
      }
      frame True {
        # "Capture Image\nImage Capture currently active, transmitting data."
        n280 = call "Image_Snap_Dual.vi"("input cluster"=w506, "Detect Movement"=w505) -> ("Framerate"=→"Framerate":i32)  [unwired: 6 in, 3 out]
      }
    }
  }
  n281 = while {
    tunnel: w2 -> [w512]
    tunnel: w3 -> [w510]
    tunnel: w2 -> [w508]
    stop <- w514 stop-if-true
    # "Image Save"
    n282 = call <extravilib>:"Read.vi"("channel"=w512) -> ("element"=w511:T4)  [unwired: 1 in, 1 out]
    n283 = call <extravilib>:"Read.vi"("channel"=w510) -> ("element"=w513:bool)  [unwired: 1 in, 1 out]
    n284 = Unbundle By Name(w511) -> ("Img_Capt"=w515:bool)
    n285 = case shown="True" w515 {
      tunnel: w510 -> [_ w522]
      tunnel: [TRUE ("Last Image?") w520] -> w509
      tunnel: w508 -> [_ w521]
      frame False {
        n286 = local write "Image Saving"(T2 {"# elements in queue"=0, "# elements in queue"=0} ("Image Saving")) -> ()
        n287 = Wait (ms)(milliseconds to wait=u32 10) -> ()  [unwired: 1 out]
      }
      frame True {
        n288 = while {
          tunnel: w522 -> [w528]
          tunnel: w521 -> [w527]
          tunnel: [w524] -> w520
          stop <- w524 stop-if-true
          n289 = call <extravilib>:"Read.vi"("channel"=w527) -> ("element"=w526:T4)  [unwired: 1 in, 1 out]
          n290 = call <extravilib>:"Read.vi"("channel"=w528) -> ("element"=w525:bool)  [unwired: 1 in, 1 out]
          n291 = call "Image_Save_Handler.vi"("Stop?"=w525, "Data"=w526) -> ("Stop out"=w524:bool, "Queue size"=→"Image Saving":T2)  [unwired: 7 in, 1 out]
        }
      }
    }
    n292 = And(x=w509, y=w513) -> (x .and. y?=w514:bool)
    n293 = case shown="True" w514 {
      frame False {
      }
      frame True {
        n294 = call "IMAQ Dispose"("All Images? (No)"=TRUE) -> ()  [unwired: 5 in, 1 out]
      }
    }
  }
